vi "KE3706A_CommandsGlobal.vi"() -> ()   [LabVIEW 2013, in "KE3706A.lvclass"]
uses:
  KE3706A.lvclass
panel:
  in  "Keithley 3706A Switching GPIB Setup":T1={"Instrument name"="Keithley 3706A", "Instrument type"=2, "Command \"Matrix Reset\""="reset()", "Command \"connect channel exclusively\""="exclusiveclose", "Command \"Disconnect all MUX Channels\""="channel.open(\"allsplots\")", "Mux1 slot"="1", "Mux2 slot"="2"} {"Instrument type" items=["Supply", "LCR", "Switching"]}
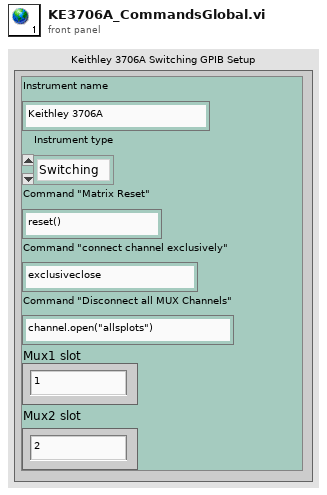
[diagram p1: front panel]
types:
  T1 = cluster{"Instrument name":string, "Instrument type":u16, "Command \"Matrix Reset\"":string, "Command \"connect channel exclusively\"":string, "Command \"Disconnect all MUX Channels\"":string, "Mux1 slot":string, "Mux2 slot":string}
diagram:
